vi "Get Index.vi"(0 "Numeric Control in":fxp<+/-,32,32>, 1 "Matrix In":fxp<+,64,57>[](array[numeric])=[0.0, 0.0, 0.0, 0.0, 0.0, 0.0, 0.0, 0.0, 0.0] format="%.25g") -> (14 "Numeric Control out":fxp<+,64,57> format="%.25g")   [LabVIEW 2014]
uses:
  <vilib>/rvi/FXPMathLib/FxpMul/XNode/nifxpmath_Multiplier.xnode
  <vilib>/rvi/FXPMathLib/FxpAdd/XNode/nifxpmath_Add.xnode
  <vilib>/rvi/FXPMathLib/sim/FxpSim.dll
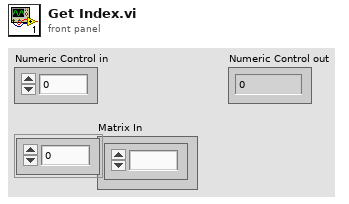
[diagram p1: front panel]
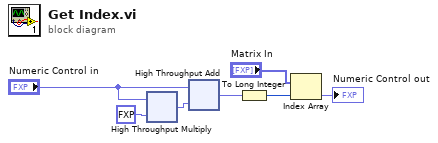
[diagram p0: block diagram]
diagram:
  n1 = xnode "High Throughput Multiply"("x"="Numeric Control in", "y"=fxp<+,2,2> 3.0 ("x")) -> ("x*y"=w1:fxp<+/-,8,8>)
  n2 = xnode "High Throughput Add"("x"="Numeric Control in", "y"=w1) -> ("x+y"=w5:fxp<+/-,8,8>)
  n3 = To Long Integer(number=w5) -> (32bit integer=w4:i32)
  n4 = Index Array(array="Matrix In", index=w4) -> (element=→"Numeric Control out":fxp<+,64,57>)
